vi "Joystick Controls.vi"() -> ()   [LabVIEW 2017]
panel:
  out "index of element":i32
  out "Boolean":bool
  out "output array 2":i32[](array[numeric])
  out "output array":i32[](array[numeric])
  out "appended array":i32[][](array[numeric])
  out "Cube Down 2":bool=TRUE
  out "Cube Up 2":bool=TRUE
  out "Deploy Ramps 2":bool=TRUE
  out "Direction Toggle 2":bool=TRUE
  in  "Button 22":bool=TRUE
  in  "Button 21":bool=TRUE
  in  "Button 20":bool=TRUE
  in  "Button 19":bool=TRUE
  in  "Button 18":bool=TRUE
  in  "Button 17":bool=TRUE
  in  "Button 16":bool=TRUE
  in  "Button 15":bool=TRUE
  in  "Button 14":bool=TRUE
  in  "Button 13":bool=TRUE
  in  "Button 12":bool=TRUE
  in  "Cube Down":bool
  in  "Cube Up":bool
  in  "Deploy Ramps":bool
  in  "Direction Toggle":bool
  in  "Gear Shift":bool
  in  "Button 11":bool
  in  "Button 10":bool
  in  "Button 9":bool
  in  "Button 8":bool
  in  "Button 7":bool
  in  "Button 6":bool
  in  "Button 5":bool
  in  "Button 4":bool
  in  "Button 3":bool
  in  "Button 2":bool
  in  "Button 1":bool
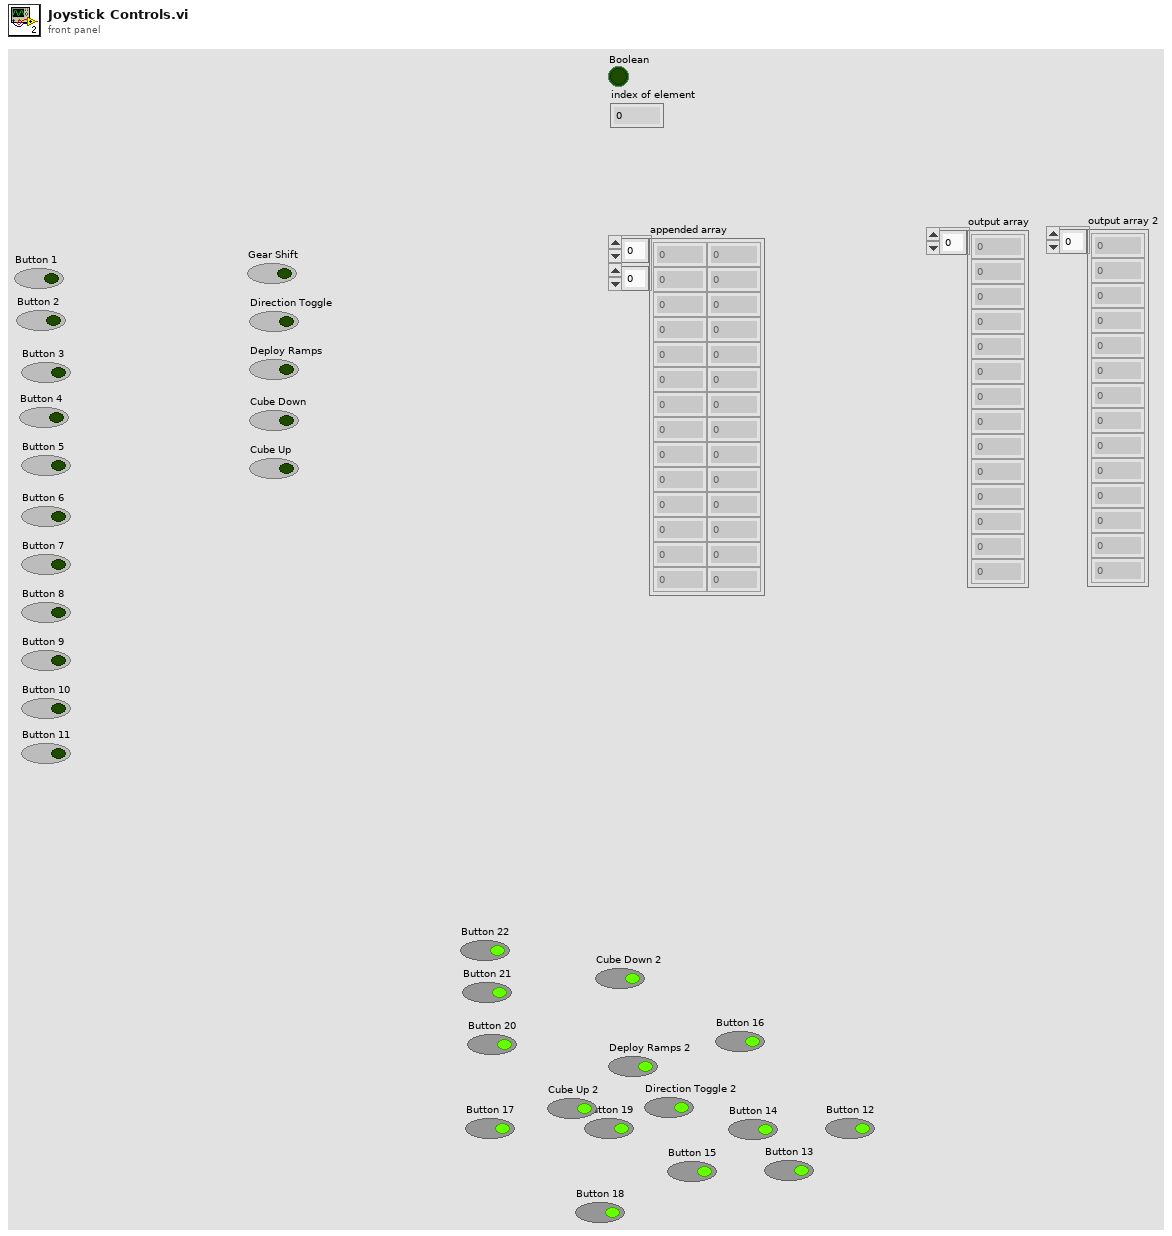
[diagram p1: front panel]
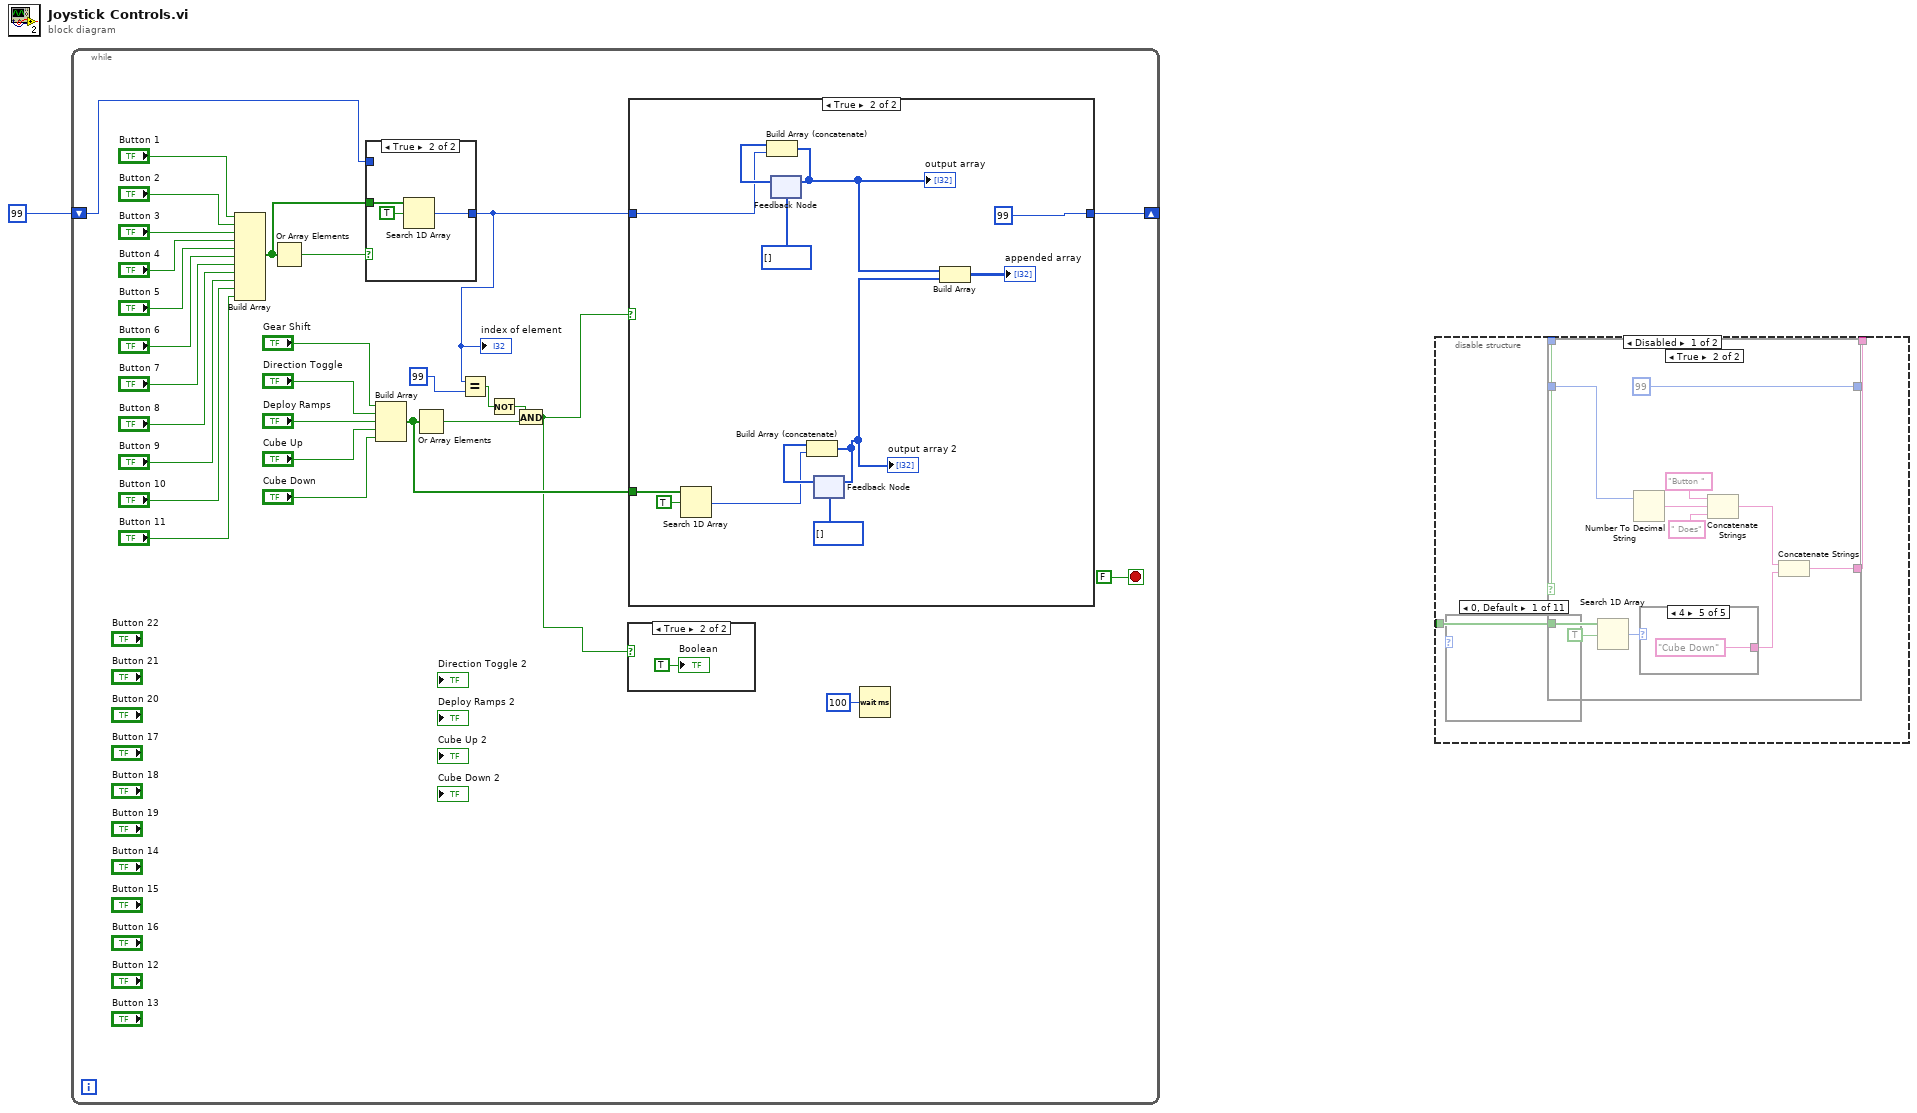
[diagram p0: block diagram]
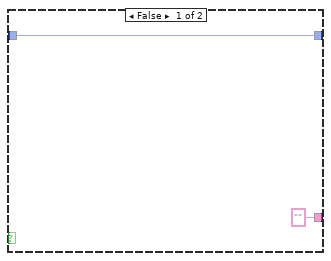
[diagram p2: hidden frame]
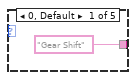
[diagram p3: hidden frame]
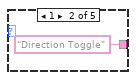
[diagram p4: hidden frame]
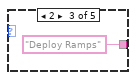
[diagram p5: hidden frame]
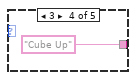
[diagram p6: hidden frame]
diagram:
  n1 = while {
    shift-right: [w6] -> _
    shift-left: 99 ("index of element") -> [w16]
    stop <- FALSE stop-if-true
    n2 = Build Array("Button 1", "Button 2", "Button 3", "Button 4", "Button 5", "Button 6", "Button 7", "Button 8", "Button 9", "Button 10", "Button 11") -> (w17:bool[])
    n3 = Or Array Elements(Boolean array=w17) -> (logical OR=w18:bool)
    n4 = case shown="True" w18 {
      tunnel: w17 -> [_ w47]
      tunnel: [w45 w46] -> w5
      tunnel: w16 -> [w45 _]
      frame False {
      }
      frame True {
        n5 = Search 1D Array(1D array=w47, element=TRUE) -> (index of element=w46:i32)  [unwired: 1 in]
      }
    }
    "index of element" <- w5
    n6 = Build Array("Gear Shift", "Direction Toggle", "Deploy Ramps", "Cube Up", "Cube Down") -> (w4:bool[])
    n7 = Or Array Elements(Boolean array=w4) -> (logical OR=w10:bool)
    n8 = Equal?(x=w5, y=99) -> (x = y?=w8:bool)
    n9 = Not(x=w8) -> (.not. x?=w9:bool)
    n10 = And(x=w9, y=w10) -> (x .and. y?=w2:bool)
    n11 = case shown="True" w2 {
      frame False {
      }
      frame True {
        "Boolean" <- TRUE
      }
    }
    n12 = case shown="True" w2 {
      tunnel: [w32 99 ("index of element")] -> w6
      tunnel: w5 -> [w32 w36]
      tunnel: w4 -> [_ w44]
      frame False {
      }
      frame True {
        n13 = Search 1D Array(1D array=w44, element=TRUE) -> (index of element=w39:i32)  [unwired: 1 in]
        n14 = feedback #1(i32[] []) -> (w37:i32[])
        n15 = Build Array (concatenate)(w37, w36) -> (w35:i32[])
        "output array" <- w35
        n16 = feedback-in #1(w35) -> ()
        n17 = feedback #2(i32[] []) -> (w40:i32[])
        n18 = Build Array (concatenate)(w40, w39) -> (w38:i32[])
        "output array 2" <- w38
        n19 = feedback-in #2(w38) -> ()
        n20 = Build Array(w35, w38) -> (→"appended array":i32[][])
      }
    }
    n21 = Wait (ms)(milliseconds to wait=u32 100) -> ()  [unwired: 1 out]
  }
  n22 = disable-structure shown="Disabled" {
    disable-tunnel: _ -> [w52 _]
    disable-tunnel: _ -> [w51 _]
    disable-tunnel: _ -> [w50 _]
    disable-tunnel: [w49 _] -> _
    frame Disabled {
      n23 = case shown="0, Default" {
        selector: _ -> [_ _ _ _ _ _ _ _ _ _ _]
        frame 0, Default {
        }
        frame 1 {
        }
        frame 2 {
        }
        frame 3 {
        }
        frame 4 {
        }
        frame 5 {
        }
        frame 6 {
        }
        frame 7 {
        }
        frame 8 {
        }
        frame 9 {
        }
        frame 10 {
        }
      }
      n24 = case shown="True" w52 {
        tunnel: w51 -> [_ w65]
        tunnel: [w54 99 ("index of element")] -> _
        tunnel: w50 -> [w54 w62]
        tunnel: ["" w55] -> w49
        frame False {
        }
        frame True {
          n25 = Search 1D Array(1D array=w65, element=TRUE) -> (index of element=w61:i32)  [unwired: 1 in]
          n26 = Number To Decimal String(number=w62) -> (decimal integer string=w58:string)  [unwired: 1 in]
          n27 = case shown="4" w61 {
            tunnel: ["Gear Shift" "Direction Toggle" "Deploy Ramps" "Cube Up" "Cube Down"] -> w56
            frame 0, Default {
            }
            frame 1 {
            }
            frame 2 {
            }
            frame 3 {
            }
            frame 4 {
            }
          }
          n28 = Concatenate Strings("Button ", w58, " Does") -> (w57:string)
          n29 = Concatenate Strings(w57, w56) -> (w55:string)
        }
      }
    }
    frame Enabled {
    }
  }
